vi "Lang Read Language File.vi"(8 "error in (no error)":errorcluster, 11 "Language Name":string) -> (0 "error out":errorcluster, 2 "Exist?":bool, 3 "UI Descriptions":T1)   [LabVIEW 2018, in "Framework.lvlib" / "Framework.lvclass"]
uses:
  Framework/Framework/Framework.lvclass
  Framework/Framework/Const Lang Setting.ctl
  Framework/Framework/Const Lang MainWnd.ctl
  Framework/Framework/Const Lang MainWnd Frame Title.ctl
  Framework/Framework/Const Lang Property.ctl
  Framework/Framework/Const Lang MainWnd Frame Basic.ctl
  Framework/Framework/Const Lang MainWnd Frame Skill.ctl
  Framework/Framework/Const Lang MainWnd Frame bp.ctl
  Framework/Framework/Const Lang MainWnd Frame w.ctl
  Framework/Framework/Const Lang MainWnd Frame b.ctl
  Framework/Framework/Const Lang MainWnd Frame i.ctl
  Framework/Framework/Const Lang MainWnd Frame o.ctl
  Framework/Framework/Const Lang MainWnd Frame c.ctl
  Framework/Framework/Const Lang MainWnd Other.ctl
  Framework/Framework/Const Lang MainWnd Menu.ctl
  Framework/Framework/Const Lang CfgWnd.ctl
  Framework/Framework/Const Lang CfgWnd Tab.ctl
  Framework/Framework/Const Lang CfgWnd Main.ctl
  Framework/Framework/Const Lang CfgWnd Path.ctl
  Framework/Framework/Const Lang CfgWnd Image.ctl
  136ff03b-022a-4f22-8316-e9f628dcce0b.vi
  <vilib>/JDP Science/JSONtext/JSON text to Variant.vi
  <vilib>/JDP Science/JSONtext/LVClass Serializer/JSONtext LVClass Serializer.lvclass
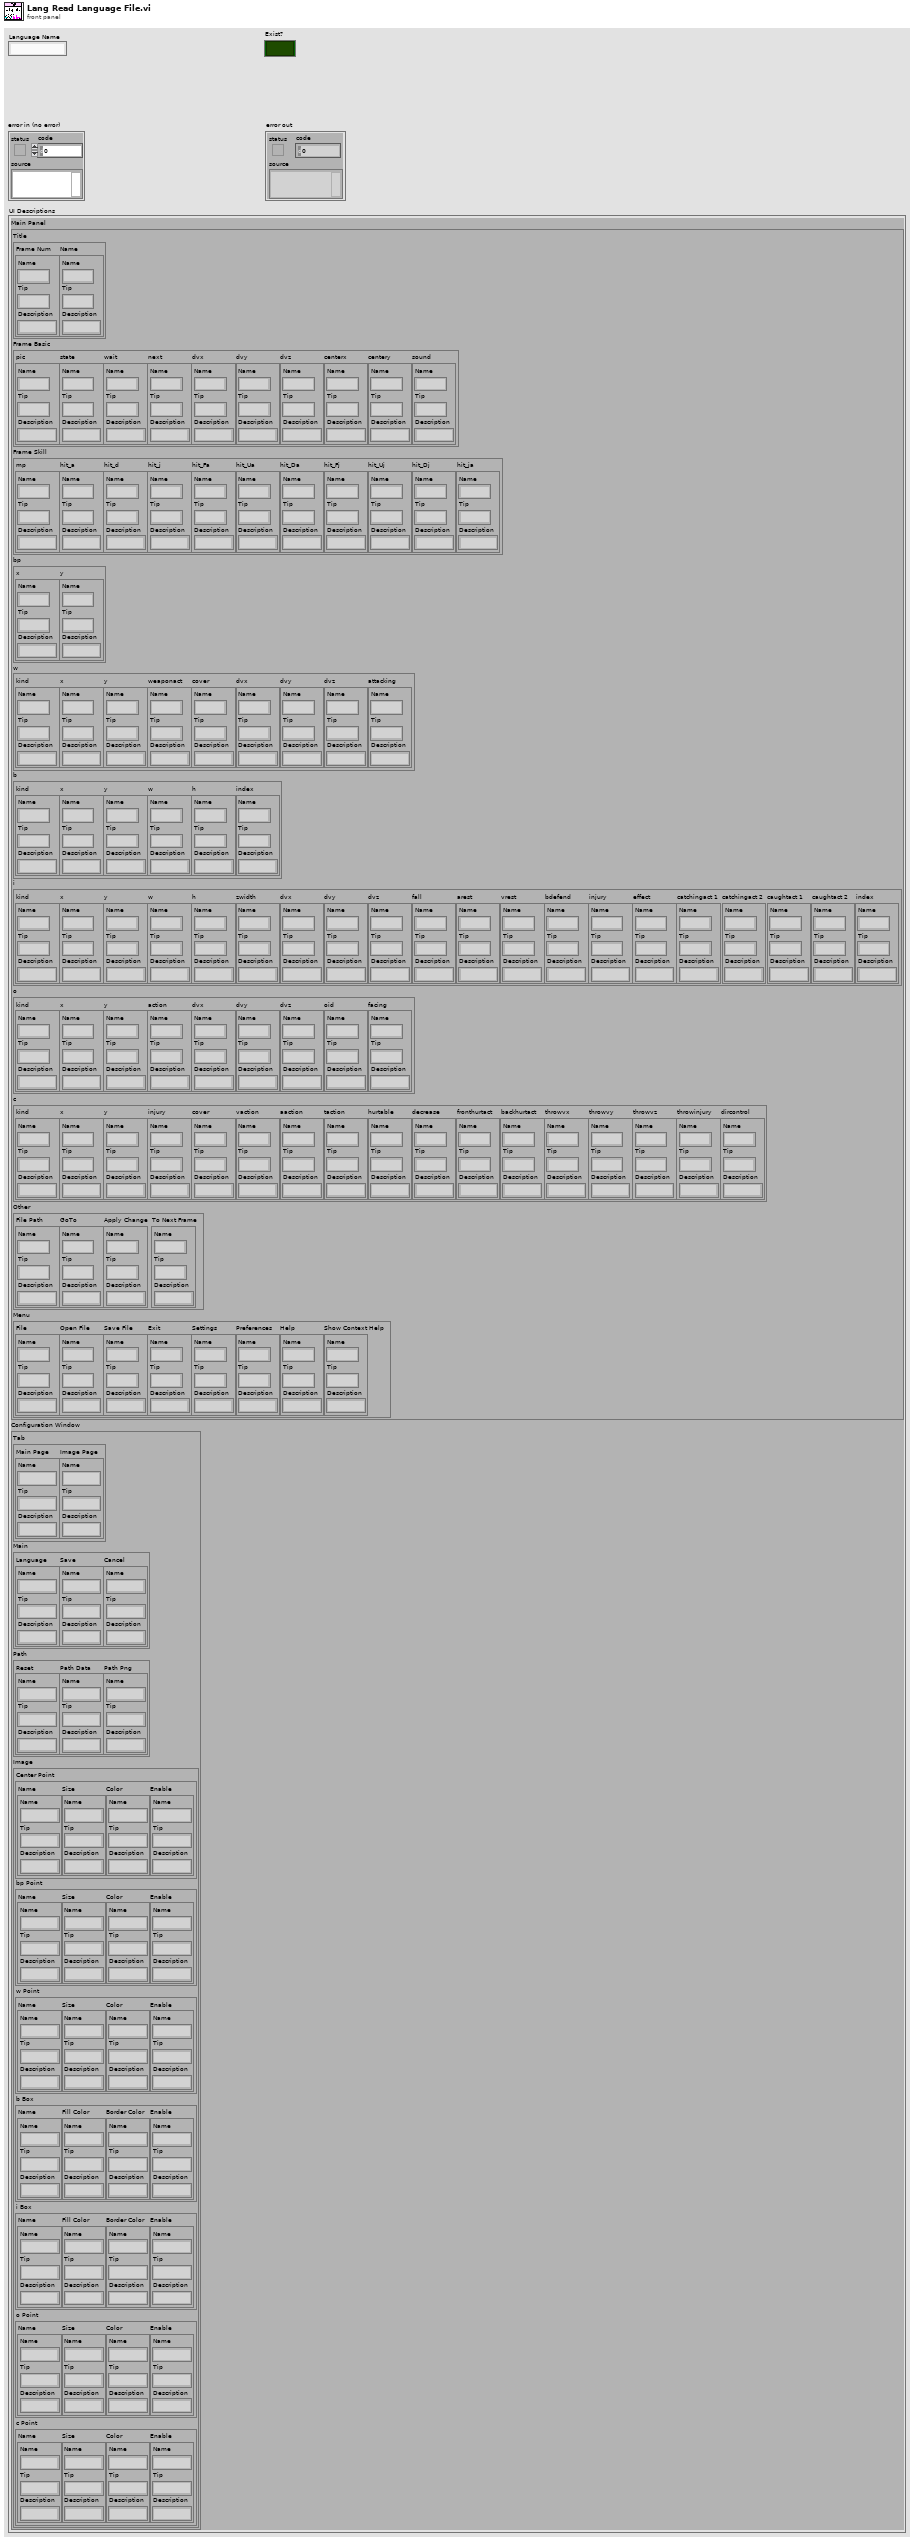
[diagram p1: front panel]
types:
  T1 = typedef "Framework.lvlib/Framework.lvclass/Const Lang Setting.ctl" = cluster{"Main Panel":T2, "Configuration Window":T15}
  T2 = typedef "Framework.lvlib/Framework.lvclass/Const Lang MainWnd.ctl" = cluster{"Title":T3, "Frame Basic":T5, "Frame Skill":T6, "bp":T7, "w":T8, "b":T9, "i":T10, "o":T11, "c":T12, "Other":T13, "Menu":T14}
  T3 = typedef "Framework.lvlib/Framework.lvclass/Const Lang MainWnd Frame Title.ctl" = cluster{"Frame Num":T4, "Name":T4}
  T4 = typedef "Framework.lvlib/Framework.lvclass/Const Lang Property.ctl" = cluster{"Name":string, "Tip":string, "Description":string}
  T5 = typedef "Framework.lvlib/Framework.lvclass/Const Lang MainWnd Frame Basic.ctl" = cluster{"pic":T4, "state":T4, "wait":T4, "next":T4, "dvx":T4, "dvy":T4, "dvz":T4, "centerx":T4, "centery":T4, "sound":T4}
  T6 = typedef "Framework.lvlib/Framework.lvclass/Const Lang MainWnd Frame Skill.ctl" = cluster{"mp":T4, "hit_a":T4, "hit_d":T4, "hit_j":T4, "hit_Fa":T4, "hit_Ua":T4, "hit_Da":T4, "hit_Fj":T4, "hit_Uj":T4, "hit_Dj":T4, "hit_ja":T4}
  T7 = typedef "Framework.lvlib/Framework.lvclass/Const Lang MainWnd Frame bp.ctl" = cluster{"x":T4, "y":T4}
  T8 = typedef "Framework.lvlib/Framework.lvclass/Const Lang MainWnd Frame w.ctl" = cluster{"kind":T4, "x":T4, "y":T4, "weaponact":T4, "cover":T4, "dvx":T4, "dvy":T4, "dvz":T4, "attacking":T4}
  T9 = typedef "Framework.lvlib/Framework.lvclass/Const Lang MainWnd Frame b.ctl" = cluster{"kind":T4, "x":T4, "y":T4, "w":T4, "h":T4, "index":T4}
  T10 = typedef "Framework.lvlib/Framework.lvclass/Const Lang MainWnd Frame i.ctl" = cluster{"kind":T4, "x":T4, "y":T4, "w":T4, "h":T4, "zwidth":T4, "dvx":T4, "dvy":T4, "dvz":T4, "fall":T4, "arest":T4, "vrest":T4, "bdefend":T4, "injury":T4, "effect":T4, "catchingact 1":T4, "catchingact 2":T4, "caughtact 1":T4, "caughtact 2":T4, "index":T4}
  T11 = typedef "Framework.lvlib/Framework.lvclass/Const Lang MainWnd Frame o.ctl" = cluster{"kind":T4, "x":T4, "y":T4, "action":T4, "dvx":T4, "dvy":T4, "dvz":T4, "oid":T4, "facing":T4}
  T12 = typedef "Framework.lvlib/Framework.lvclass/Const Lang MainWnd Frame c.ctl" = cluster{"kind":T4, "x":T4, "y":T4, "injury":T4, "cover":T4, "vaction":T4, "aaction":T4, "taction":T4, "hurtable":T4, "decrease":T4, "fronthurtact":T4, "backhurtact":T4, "throwvx":T4, "throwvy":T4, "throwvz":T4, "throwinjury":T4, "dircontrol":T4}
  T13 = typedef "Framework.lvlib/Framework.lvclass/Const Lang MainWnd Other.ctl" = cluster{"File Path":T4, "GoTo":T4, "Apply Change":T4, "To Next Frame":T4}
  T14 = typedef "Framework.lvlib/Framework.lvclass/Const Lang MainWnd Menu.ctl" = cluster{"File":T4, "Open File":T4, "Save File":T4, "Exit":T4, "Settings":T4, "Preferences":T4, "Help":T4, "Show Context Help":T4}
  T15 = typedef "Framework.lvlib/Framework.lvclass/Const Lang CfgWnd.ctl" = cluster{"Tab":T16, "Main":T17, "Path":T18, "Image":T19}
  T16 = typedef "Framework.lvlib/Framework.lvclass/Const Lang CfgWnd Tab.ctl" = cluster{"Main Page":T4, "Image Page":T4}
  T17 = typedef "Framework.lvlib/Framework.lvclass/Const Lang CfgWnd Main.ctl" = cluster{"Language":T4, "Save":T4, "Cancel":T4}
  T18 = typedef "Framework.lvlib/Framework.lvclass/Const Lang CfgWnd Path.ctl" = cluster{"Reset":T4, "Path Data":T4, "Path Png":T4}
  T19 = typedef "Framework.lvlib/Framework.lvclass/Const Lang CfgWnd Image.ctl" = cluster{"Center Point":cluster{"Name":T4, "Size":T4, "Color":T4, "Enable":T4}, "bp Point":cluster{"Name":T4, "Size":T4, "Color":T4, "Enable":T4}, "w Point":cluster{"Name":T4, "Size":T4, "Color":T4, "Enable":T4}, "b Box":cluster{"Name":T4, "Fill Color":T4, "Border Color":T4, "Enable":T4}, "i Box":cluster{"Name":T4, "Fill Color":T4, "Border Color":T4, "Enable":T4}, "o Point":cluster{"Name":T4, "Size":T4, "Color":T4, "Enable":T4}, "c Point":cluster{"Name":T4, "Size":T4, "Color":T4, "Enable":T4}}
  T20 = enum16{"open", "replace", "create", "open or create", "replace or create", "replace or create with confirmation"}
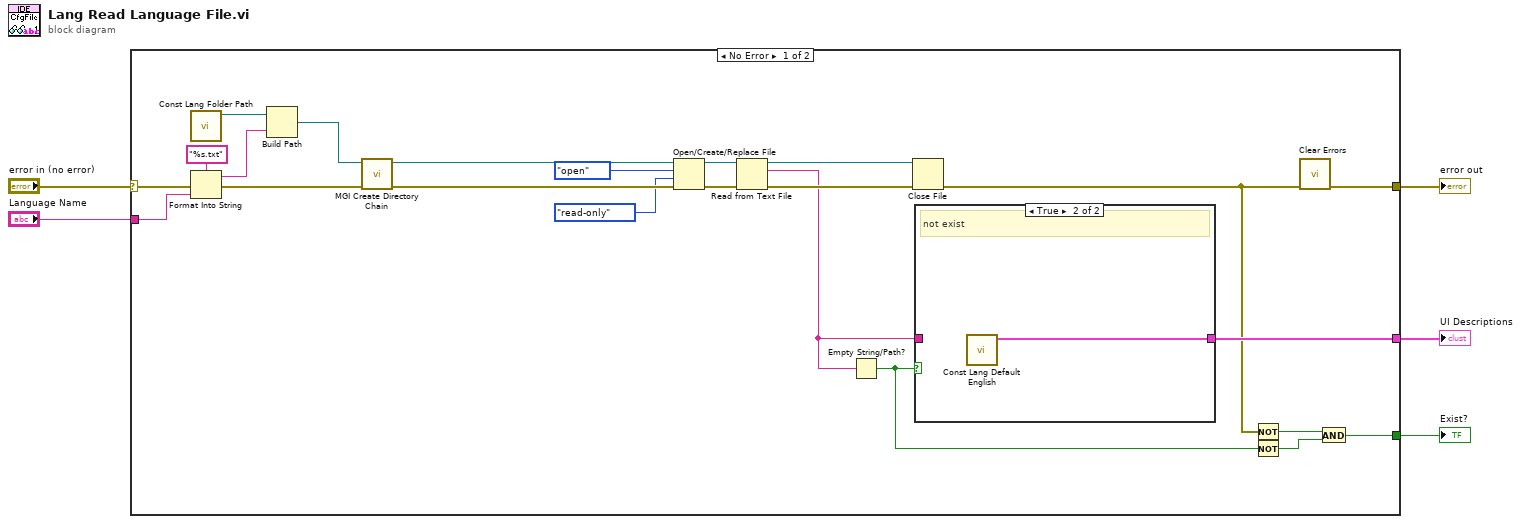
[diagram p0: block diagram]
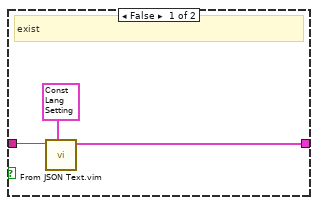
[diagram p2: hidden frame]
diagram:
  n1 = case shown="No Error" "error in (no error)" {
    selector: "error in (no error)" -> [w8 w33]
    tunnel: [w18 w33] -> w4
    tunnel: [w19 _] -> w1
    tunnel: [w15 _] -> w3
    tunnel: "Language Name" -> [w11 _]
    frame No Error {
      n2 = call "Const Lang Folder Path.vi"() -> ("Language Folder Path"=w12:path)  [unwired: 11 in]
      n3 = Format Into String(format string="%s.txt", error in=w8, w11) -> (resulting string=w9:string, error out=w7:errorcluster)  [unwired: 1 in]
      n4 = Build Path(base path=w12, name or relative path=w9) -> (appended path=w6:path)
      n5 = call <userlib>:"MGI Create Directory Chain.vi"("Error In"=w7, "Path"=w6) -> ("Error Out"=w27:errorcluster, "Duplicate Path"=w28:path)  [unwired: 8 in]
      n6 = Open/Create/Replace File(file path (use dialog)=w28, error in=w27, operation (0:open)=T20."open", access (0:read/write)=enum16{"read/write", "read-only", "write-only"}."read-only") -> (refnum out=w26:refnum<file>, error out=w25:errorcluster)  [unwired: 2 in, 1 out]
      n7 = Read from Text File(file (use dialog)=w26, error in=w25) -> (refnum out=w24:refnum<file>, text=w20:string, error out=w22:errorcluster)  [unwired: 2 in, 1 out]
      n8 = Empty String/Path?(string/path=w20) -> (empty?=w17:bool)
      n9 = Close File(refnum=w24, error in=w22) -> (error out=w13:errorcluster)  [unwired: 1 out]
      n10 = case shown="True" w17 {
        tunnel: [w30 w32] -> w19
        tunnel: w20 -> [w31 _]
        frame False {
          # "exist"
          n11 = call "From JSON Text.vim"("Data Type and Default Value"=T1 {"Main Panel"={"Title"={"Frame Num"={"Name"="", "Tip"="", "Description"=""}, "Name"={"Name"="", "Tip"="", "Description"=""}}, "Frame Basic"={"pic"={"Name"="", "Tip"="", "Description"=""}, "state"={"Name"="", "Tip"="", "Description"=""}, "wait"={"Name"="", "Tip"="", "Description"=""}, "next"={"Name"="", "Tip"="", "Description"=""}, "dvx"={"Name"="", "Tip"="", "Description"=""}, "dvy"={"Name"="", "Tip"="", "Description"=""}, "dvz"={"Name"="", "Tip"="", "Description"=""}, "centerx"={"Name"="", "Tip"="", "Description"=""}, "centery"={"Name"="", "Tip"="", "Description"=""}, "sound"={"Name"="", "Tip"="", "Description"=""}}, "Frame Skill"={"mp"={"Name"="", "Tip"="", "Description"=""}, "hit_a"={"Name"="", "Tip"="", "Description"=""}, "hit_d"={"Name"="", "Tip"="", "Description"=""}, "hit_j"={"Name"="", "Tip"="", "Description"=""}, "hit_Fa"={"Name"="", "Tip"="", "Description"=""}, "hit_Ua"={"Name"="", "Tip"="", "Description"=""}, "hit_Da"={"Name"="", "Tip"="", "Description"=""}, "hit_Fj"={"Name"="", "Tip"="", "Description"=""}, "hit_Uj"={"Name"="", "Tip"="", "Description"=""}, "hit_Dj"={"Name"="", "Tip"="", "Description"=""}, "hit_ja"={"Name"="", "Tip"="", "Description"=""}}, "bp"={"x"={"Name"="", "Tip"="", "Description"=""}, "y"={"Name"="", "Tip"="", "Description"=""}}, "w"={"kind"={"Name"="", "Tip"="", "Description"=""}, "x"={"Name"="", "Tip"="", "Description"=""}, "y"={"Name"="", "Tip"="", "Description"=""}, "weaponact"={"Name"="", "Tip"="", "Description"=""}, "cover"={"Name"="", "Tip"="", "Description"=""}, "dvx"={"Name"="", "Tip"="", "Description"=""}, "dvy"={"Name"="", "Tip"="", "Description"=""}, "dvz"={"Name"="", "Tip"="", "Description"=""}, "attacking"={"Name"="", "Tip"="", "Description"=""}}, "b"={"kind"={"Name"="", "Tip"="", "Description"=""}, "x"={"Name"="", "Tip"="", "Description"=""}, "y"={"Name"="", "Tip"="", "Description"=""}, "w"={"Name"="", "Tip"="", "Description"=""}, "h"={"Name"="", "Tip"="", "Description"=""}, "index"={"Name"="", "Tip"="", "Description"=""}}, "i"={"kind"={"Name"="", "Tip"="", "Description"=""}, "x"={"Name"="", "Tip"="", "Description"=""}, "y"={"Name"="", "Tip"="", "Description"=""}, "w"={"Name"="", "Tip"="", "Description"=""}, "h"={"Name"="", "Tip"="", "Description"=""}, "zwidth"={"Name"="", "Tip"="", "Description"=""}, "dvx"={"Name"="", "Tip"="", "Description"=""}, "dvy"={"Name"="", "Tip"="", "Description"=""}, "dvz"={"Name"="", "Tip"="", "Description"=""}, "fall"={"Name"="", "Tip"="", "Description"=""}, "arest"={"Name"="", "Tip"="", "Description"=""}, "vrest"={"Name"="", "Tip"="", "Description"=""}, "bdefend"={"Name"="", "Tip"="", "Description"=""}, "injury"={"Name"="", "Tip"="", "Description"=""}, "effect"={"Name"="", "Tip"="", "Description"=""}, "catchingact 1"={"Name"="", "Tip"="", "Description"=""}, "catchingact 2"={"Name"="", "Tip"="", "Description"=""}, "caughtact 1"={"Name"="", "Tip"="", "Description"=""}, "caughtact 2"={"Name"="", "Tip"="", "Description"=""}, "index"={"Name"="", "Tip"="", "Description"=""}}, "o"={"kind"={"Name"="", "Tip"="", "Description"=""}, "x"={"Name"="", "Tip"="", "Description"=""}, "y"={"Name"="", "Tip"="", "Description"=""}, "action"={"Name"="", "Tip"="", "Description"=""}, "dvx"={"Name"="", "Tip"="", "Description"=""}, "dvy"={"Name"="", "Tip"="", "Description"=""}, "dvz"={"Name"="", "Tip"="", "Description"=""}, "oid"={"Name"="", "Tip"="", "Description"=""}, "facing"={"Name"="", "Tip"="", "Description"=""}}, "c"={"kind"={"Name"="", "Tip"="", "Description"=""}, "x"={"Name"="", "Tip"="", "Description"=""}, "y"={"Name"="", "Tip"="", "Description"=""}, "injury"={"Name"="", "Tip"="", "Description"=""}, "cover"={"Name"="", "Tip"="", "Description"=""}, "vaction"={"Name"="", "Tip"="", "Description"=""}, "aaction"={"Name"="", "Tip"="", "Description"=""}, "taction"={"Name"="", "Tip"="", "Description"=""}, "hurtable"={"Name"="", "Tip"="", "Description"=""}, "decrease"={"Name"="", "Tip"="", "Description"=""}, "fronthurtact"={"Name"="", "Tip"="", "Description"=""}, "backhurtact"={"Name"="", "Tip"="", "Description"=""}, "throwvx"={"Name"="", "Tip"="", "Description"=""}, "throwvy"={"Name"="", "Tip"="", "Description"=""}, "throwvz"={"Name"="", "Tip"="", "Description"=""}, "throwinjury"={"Name"="", "Tip"="", "Description"=""}, "dircontrol"={"Name"="", "Tip"="", "Description"=""}}, "Other"={"File Path"={"Name"="", "Tip"="", "Description"=""}, "GoTo"={"Name"="", "Tip"="", "Description"=""}, "Apply Change"={"Name"="", "Tip"="", "Description"=""}, "To Next Frame"={"Name"="", "Tip"="", "Description"=""}}, "Menu"={"File"={"Name"="", "Tip"="", "Description"=""}, "Open File"={"Name"="", "Tip"="", "Description"=""}, "Save File"={"Name"="", "Tip"="", "Description"=""}, "Exit"={"Name"="", "Tip"="", "Description"=""}, "Settings"={"Name"="", "Tip"="", "Description"=""}, "Preferences"={"Name"="", "Tip"="", "Description"=""}, "Help"={"Name"="", "Tip"="", "Description"=""}, "Show Context Help"={"Name"="", "Tip"="", "Description"=""}}}, "Configuration Window"={"Tab"={"Main Page"={"Name"="", "Tip"="", "Description"=""}, "Image Page"={"Name"="", "Tip"="", "Description"=""}}, "Main"={"Language"={"Name"="", "Tip"="", "Description"=""}, "Save"={"Name"="", "Tip"="", "Description"=""}, "Cancel"={"Name"="", "Tip"="", "Description"=""}}, "Path"={"Reset"={"Name"="", "Tip"="", "Description"=""}, "Path Data"={"Name"="", "Tip"="", "Description"=""}, "Path Png"={"Name"="", "Tip"="", "Description"=""}}, "Image"={"Center Point"={"Name"={"Name"="", "Tip"="", "Description"=""}, "Size"={"Name"="", "Tip"="", "Description"=""}, "Color"={"Name"="", "Tip"="", "Description"=""}, "Enable"={"Name"="", "Tip"="", "Description"=""}}, "bp Point"={"Name"={"Name"="", "Tip"="", "Description"=""}, "Size"={"Name"="", "Tip"="", "Description"=""}, "Color"={"Name"="", "Tip"="", "Description"=""}, "Enable"={"Name"="", "Tip"="", "Description"=""}}, "w Point"={"Name"={"Name"="", "Tip"="", "Description"=""}, "Size"={"Name"="", "Tip"="", "Description"=""}, "Color"={"Name"="", "Tip"="", "Description"=""}, "Enable"={"Name"="", "Tip"="", "Description"=""}}, "b Box"={"Name"={"Name"="", "Tip"="", "Description"=""}, "Fill Color"={"Name"="", "Tip"="", "Description"=""}, "Border Color"={"Name"="", "Tip"="", "Description"=""}, "Enable"={"Name"="", "Tip"="", "Description"=""}}, "i Box"={"Name"={"Name"="", "Tip"="", "Description"=""}, "Fill Color"={"Name"="", "Tip"="", "Description"=""}, "Border Color"={"Name"="", "Tip"="", "Description"=""}, "Enable"={"Name"="", "Tip"="", "Description"=""}}, "o Point"={"Name"={"Name"="", "Tip"="", "Description"=""}, "Size"={"Name"="", "Tip"="", "Description"=""}, "Color"={"Name"="", "Tip"="", "Description"=""}, "Enable"={"Name"="", "Tip"="", "Description"=""}}, "c Point"={"Name"={"Name"="", "Tip"="", "Description"=""}, "Size"={"Name"="", "Tip"="", "Description"=""}, "Color"={"Name"="", "Tip"="", "Description"=""}, "Enable"={"Name"="", "Tip"="", "Description"=""}}}}} ("UI Descriptions"), "JSON"=w31) -> ("Data out"=w30:T1)  [unwired: 8 in, 1 out]
        }
        frame True {
          # "not exist"
          n12 = call "Const Lang Default English.vi"() -> ("UI Descriptions"=w32:T1)  [unwired: 11 in]
        }
      }
      n13 = Not(x=w13) -> (.not. x?=w16:bool)
      n14 = Not(x=w17) -> (.not. x?=w14:bool)
      n15 = call <vilib>:"Clear Errors.vi"("error in (no error)"=w13) -> ("error out"=w18:errorcluster)  [unwired: 5 in, 1 out]
      n16 = And(x=w16, y=w14) -> (x .and. y?=w15:bool)
    }
    frame Error {
    }
  }
  "error out" <- w4
  "Exist?" <- w3
  "UI Descriptions" <- w1
